vi "dequeue.vi"(8 "error in (no error)":errorcluster, 11 "EventDaemon in":refnum<class "TemplateDaemon.lvclass">) -> (0 "error out":errorcluster, 2 "state":T1, 3 "EventDaemon out":refnum<class "TemplateDaemon.lvclass">, 5 "timeout":i32)   [LabVIEW 2020, in "TemplateDaemon.lvclass"]
doc: "Dequeues private states for daemon."
uses:
  TemplateDaemon.lvclass
  states--enum.ctl
  TemplateDaemon.lvclass/TemplateDaemon.ctl
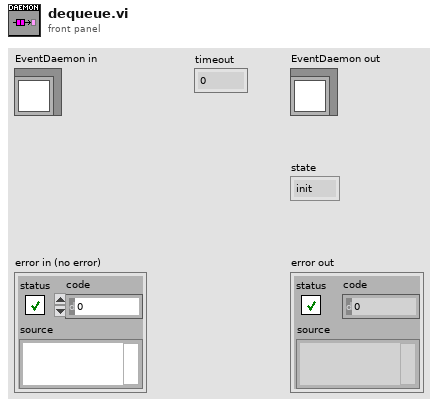
[diagram p1: front panel]
types:
  T1 = typedef "TemplateDaemon.lvclass/states--enum.ctl" = enum16{"init", "default", "error handler", "exit"}
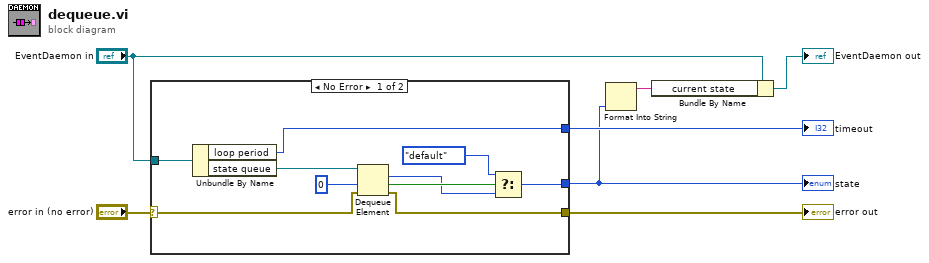
[diagram p0: block diagram]
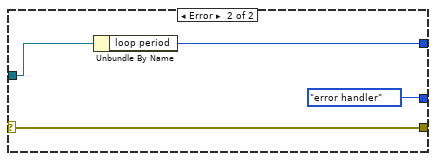
[diagram p2: hidden frame]
diagram:
  n1 = case shown="No Error" "error in (no error)" {
    selector: "error in (no error)" -> [w9 w20]
    tunnel: "EventDaemon in" -> [w17 w19]
    tunnel: [w14 w20] -> w7
    tunnel: [w10 states--enum."error handler" ("states")] -> w1
    tunnel: [w8 w18] -> w5
    frame No Error {
      n2 = Unbundle By Name(w17) -> ("loop period"=w8:i32, "state queue"=w16:refnum<queue>)
      n3 = Dequeue Element(queue=w16, timeout in ms (-1)=0, error in (no error)=w9) -> (element=w12:T1, timed out?=w13:bool, error out=w14:errorcluster)  [unwired: 1 out]
      n4 = Select(t=states--enum."default", s=w13, f=w12) -> (s? t:f=w10:T1)
    }
    frame Error {
      n5 = Unbundle By Name(w19) -> ("loop period"=w18:i32)
    }
  }
  "error out" <- w7
  "state" <- w1
  "timeout" <- w5
  n6 = Format Into String(w1) -> (resulting string=w2:string)  [unwired: 3 in, 1 out]
  n7 = Bundle By Name(cluster="EventDaemon in", "current state"=w2) -> (→"EventDaemon out":refnum<class "TemplateDaemon.lvclass">)
